vi "gather and display vision.vi"(7 "intensity plot in":i32[][](array[numeric]), 8 "error in (no error)":errorcluster, 9 "Energy 2d gate":T1, 10 "which spectrum":string) -> (0 "error out":errorcluster, 1 "Y Axis":string, 2 "X Axis":string, 5 "intensity plot out":i32[][](array[numeric]))   [LabVIEW 2016]
doc: "This vi takes the gated region values from the pixie and allows the user to select which \nspectrum to view."
uses:
  controls/energy 2d selection.ctl
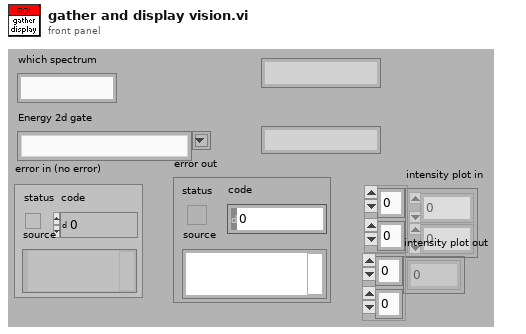
[diagram p1: front panel]
types:
  T1 = typedef "energy 2d selection.ctl" = string
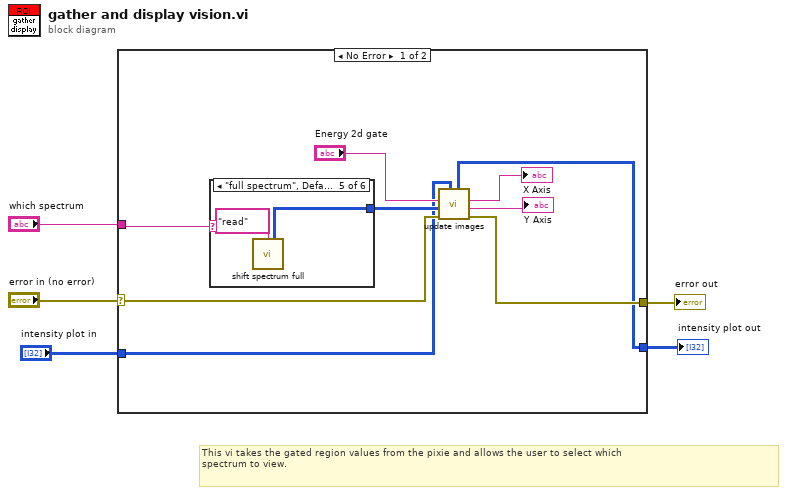
[diagram p0: block diagram]
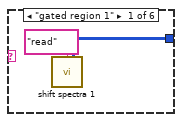
[diagram p2: hidden frame]
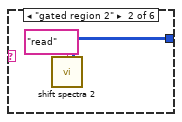
[diagram p3: hidden frame]
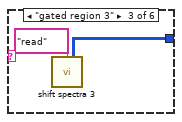
[diagram p4: hidden frame]
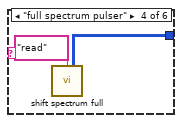
[diagram p5: hidden frame]
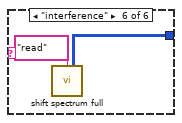
[diagram p6: hidden frame]
diagram:
  # "This vi takes the gated region values from the pixie and allows the user to select which \nspectrum to view."
  n1 = case shown="No Error" "error in (no error)" {
    selector: "error in (no error)" -> [w9 w28]
    tunnel: "which spectrum" -> [w13 _]
    tunnel: [w11 w28] -> w4
    tunnel: [w8 w27] -> w2
    tunnel: "intensity plot in" -> [w7 w27]
    frame No Error {
      n2 = case shown="\"full spectrum\", Default" w13 {
        tunnel: [w15 w17 w19 w21 w23 w25] -> w12
        frame "gated region 1" {
          n3 = call "shift spectra 1.vi"("shift control"="read") -> ("2d intensity array output"=w15:i32[][])  [unwired: 8 in, 6 out]
        }
        frame "gated region 2" {
          n4 = call "shift spectra 2.vi"("shift control"="read") -> ("2d intensity array output"=w17:i32[][])  [unwired: 8 in, 6 out]
        }
        frame "gated region 3" {
          n5 = call "shift spectra 3.vi"("shift control"="read") -> ("2d intensity array output"=w19:i32[][])  [unwired: 8 in, 6 out]
        }
        frame "full spectrum pulser" {
          n6 = call "shift spectrum full.vi"("shift control"="read") -> ("2d intensity array output"=w21:i32[][])  [unwired: 8 in, 6 out]
        }
        frame "full spectrum", Default {
          n7 = call "shift spectrum full.vi"("shift control"="read") -> ("2d intensity array output"=w23:i32[][])  [unwired: 8 in, 6 out]
        }
        frame "interference" {
          n8 = call "shift spectrum full.vi"("shift control"="read") -> ("2d intensity array output"=w25:i32[][])  [unwired: 8 in, 6 out]
        }
      }
      n9 = call "update images.vi"("intensity plot in"=w7, "error in (no error)"=w9, "realtime data input"=w12, "Energy 2d gate"="Energy 2d gate") -> ("error out"=w11:errorcluster, "Y name"=→"Y Axis":string, "X name"=→"X Axis":string, "intensity plot out"=w8:i32[][])  [unwired: 4 in]
    }
    frame Error {
    }
  }
  "error out" <- w4
  "intensity plot out" <- w2
